vi "Get SD Normal Mode Channels.vi"(8 "error in (no error)":errorcluster, 11 "9401 in":refnum<class "9401.lvclass">) -> (0 "error out":errorcluster, 1 "Channels":T2, 2 "Channel Names":string[](array[string]), 3 "9401 out":refnum<class "9401.lvclass">, 4 "Type":T1)   [LabVIEW 2017, in "Modules.lvlib" / "9401.lvclass"]
uses:
  9401.lvclass
  RSI Module/Channels.ctl
  RSI Module/Channel Type.ctl
  <vilib>/NI Veristand/Custom Device API/Custom Device Channel Type.ctl
  9401.lvclass/9401.ctl
  RSI Module/RSI Module.lvclass
  <vilib>/NI Veristand/Custom Device API/Custom Device API.lvlib
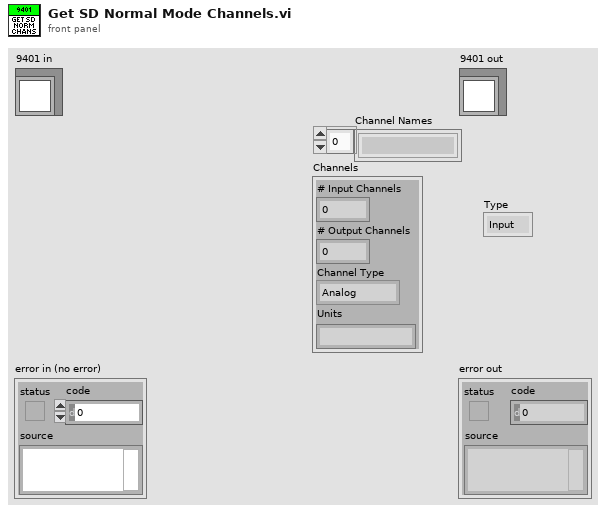
[diagram p1: front panel]
types:
  T1 = typedef "Custom Device API.lvlib/Custom Device Channel Type.ctl" = enum16{"Input", "Output"}
  T2 = typedef "Modules.lvlib/RSI Module.lvclass/Channels.ctl" = cluster{"# Input Channels":i32, "# Output Channels":i32, "Channel Type":T3, "Units":string}
  T3 = typedef "Modules.lvlib/RSI Module.lvclass/Channel Type.ctl" = enum16{"Analog", "Digital"}
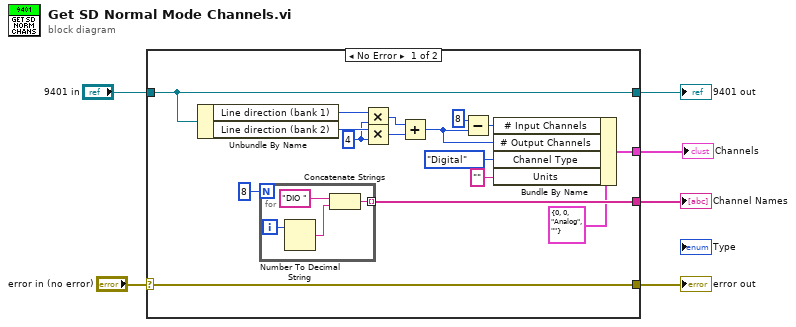
[diagram p0: block diagram]
diagram:
  n1 = case shown="No Error" "error in (no error)" {
    selector: "error in (no error)" -> [w20 w28]
    tunnel: [w20 w28] -> w5
    tunnel: "9401 in" -> [w19 w27]
    tunnel: [w19 w27] -> w3
    tunnel: [w21 _] -> w2
    tunnel: [w7 _] -> w1
    frame No Error {
      w15 = u32 4 ("y")
      n2 = Unbundle By Name(w19) -> ("Line direction (bank 1)"=w16:u32, "Line direction (bank 2)"=w17:u32)
      n3 = for {
        N: 8 -> [_]
        tunnel: [w23] -> w21 mode=indexing
        i -> [w26]
        n4 = Number To Decimal String(number=w26) -> (decimal integer string=w24:string)  [unwired: 1 in]
        n5 = Concatenate Strings("DIO ", w24) -> (w23:string)
      }
      n6 = Multiply(x=w16, y=w15) -> (x*y=w14:u32)
      n7 = Multiply(x=w17, y=w15) -> (x*y=w13:u32)
      n8 = Add(x=w14, y=w13) -> (x+y=w11:u32)
      n9 = Subtract(x=u32 8 ("y"), y=w11) -> (x-y=w12:u32)
      n10 = Bundle By Name(cluster=T2 {"# Input Channels"=0, "# Output Channels"=0, "Channel Type"=enum."Analog", "Units"=""} ("Channels"), "# Input Channels"=w12, "# Output Channels"=w11, "Channel Type"=Channel_Type."Digital", "Units"="") -> (w7:T2)
    }
    frame Error {
    }
  }
  "error out" <- w5
  "9401 out" <- w3
  "Channel Names" <- w2
  "Channels" <- w1
